vi "Get TDMS channel with scaling.vi"(6 "Samples per read":i64=1000000, 7 "Clip/desimate":T1={"Clip time"=FALSE, "Tiime 0"=0.0, "Time 1"=0.0, "Maximum data points"=1, "Decimation method"=enum."Min-Max"}, 8 "error in":errorcluster, 9 "Channel name":string, 10 "group name":string, 11 "tdms file":refnum<k34>) -> (0 "error out":errorcluster, 1 "output waveform":waveform(dbl), 3 "tdms file out":refnum<k34>)   [LabVIEW 2015]
uses:
  Controls/Data reduction.ctl
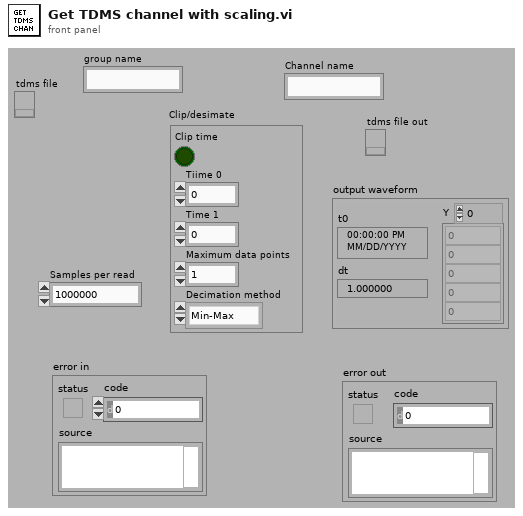
[diagram p1: front panel]
types:
  T1 = typedef "Data reduction.ctl" = cluster{"Clip time":bool, "Tiime 0":dbl, "Time 1":dbl, "Maximum data points":i32, "Decimation method":enum16{"coerce", "linear", "spline", "Min-Max", "Average"}}
  T2 = enum16{"coerce", "linear", "spline", "Min-Max", "Average"}
  T3 = typedef "TDMS channel info.ctl" = cluster{"t0":timestamp, "dt":dbl, "Channel length":i64}
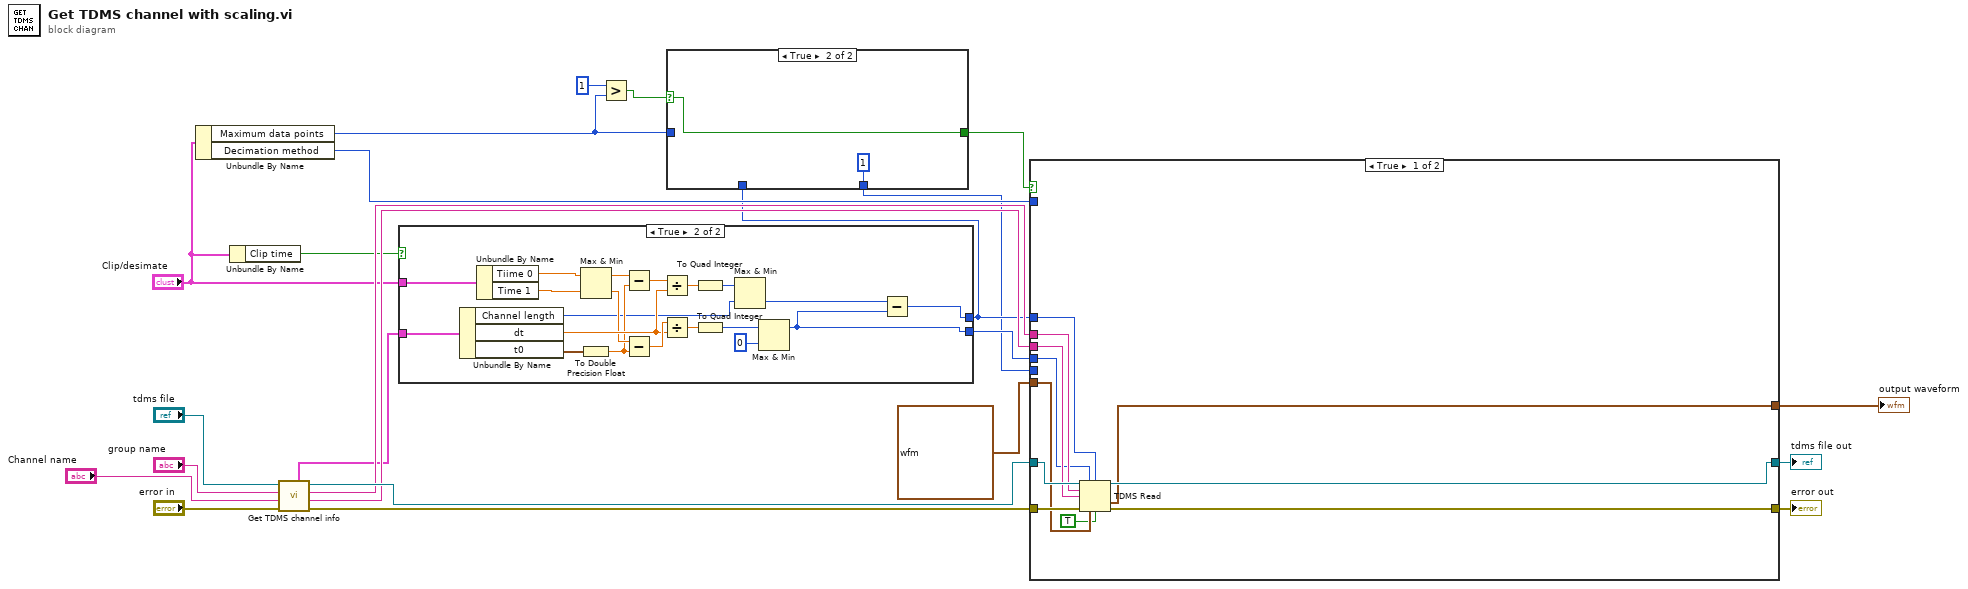
[diagram p0: block diagram]
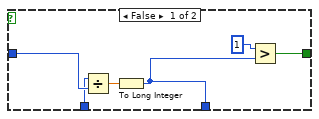
[diagram p2: hidden frame]
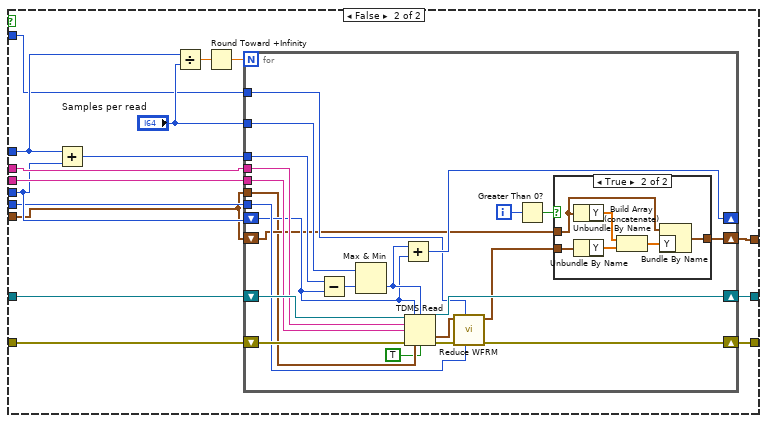
[diagram p3: hidden frame]
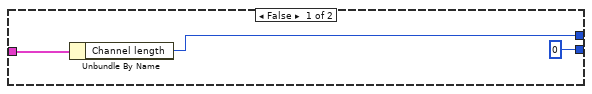
[diagram p5: hidden frame]
diagram:
  n1 = Unbundle By Name("Clip/desimate") -> ("Maximum data points"=w2:i32, "Decimation method"=w10:T2)
  n2 = Unbundle By Name("Clip/desimate") -> ("Clip time"=w7:bool)
  n3 = call "Get TDMS channel info.vi"("error in"="error in", "Channel name"="Channel name", "group name"="group name", "tdms file"="tdms file") -> ("error out"=w19:errorcluster, "channel name out"=w16:string, "group name out"=w17:string, "tdms file out"=w18:refnum<k34>, "TDMS channel info"=w6:T3)  [unwired: 3 in]
  n4 = case shown="True" w7 {
    tunnel: w6 -> [w25 w46]
    tunnel: [i64 0 ("offset (0)") w29] -> w13
    tunnel: [w24 w28] -> w4
    tunnel: "Clip/desimate" -> [_ w37]
    frame False {
      n5 = Unbundle By Name(w25) -> ("Channel length"=w24:i64)
    }
    frame True {
      n6 = Unbundle By Name(w46) -> ("Channel length"=w27:i64, "dt"=w38:dbl, "t0"=w33:timestamp)
      n7 = Unbundle By Name(w37) -> ("Tiime 0"=w36:dbl, "Time 1"=w35:dbl)
      n8 = Max & Min(x=w36, y=w35) -> (max(x,y)=w34:dbl, min(x,y)=w32:dbl)
      n9 = To Double Precision Float(number=w33) -> (double precision float=w31:dbl)
      n10 = Subtract(x=w34, y=w31) -> (x-y=w45:dbl)
      n11 = Subtract(x=w32, y=w31) -> (x-y=w44:dbl)
      n12 = Divide(x=w45, y=w38) -> (x/y=w43:dbl)
      n13 = Divide(x=w44, y=w38) -> (x/y=w40:dbl)
      n14 = To Quad Integer(1:w43) -> (0:w42:i64)
      n15 = To Quad Integer(1:w40) -> (0:w41:i64)
      n16 = Max & Min(x=w42, y=w27) -> (min(x,y)=w30:i64)  [unwired: 1 out]
      n17 = Max & Min(x=w41, y=i64 0) -> (max(x,y)=w29:i64)  [unwired: 1 out]
      n18 = Subtract(x=w30, y=w29) -> (x-y=w28:i64)
    }
  }
  n19 = Greater?(x=1 ("y"), y=w2) -> (0:w5:bool)
  n20 = case shown="True" w5 {
    selector: w5 -> [_ w54]
    tunnel: [w52 w54] -> w12
    tunnel: w2 -> [w49 _]
    tunnel: w4 -> [w48 _]
    tunnel: [w47 1] -> w1
    frame False {
      n21 = Divide(x=w48, y=w49) -> (x/y=w50:dbl)
      n22 = To Long Integer(number=w50) -> (32bit integer=w47:i32)
      n23 = Greater?(x=1 ("y"), y=w47) -> (0:w52:bool)
    }
    frame True {
    }
  }
  n24 = case shown="True" w12 {
    tunnel: w19 -> [w65 w81]
    tunnel: w18 -> [w64 w80]
    tunnel: w17 -> [w63 w79]
    tunnel: w16 -> [w62 w78]
    tunnel: [w61 w77] -> w15
    tunnel: [w60 w76] -> w14
    tunnel: w13 -> [w59 w72]
    tunnel: w4 -> [w58 w71]
    tunnel: [w57 w75] -> w11
    tunnel: w1 -> [_ w69]
    tunnel: w10 -> [_ w67]
    tunnel: waveform(dbl) {"t0"=timestamp(0 s since 1904-01-01), "dt"=1.0, "Y"=[]} ("Waveform out") -> [w56 w66]
    frame True {
      n25 = TDMS Read(0:w64, 1:w59, 2:w58, 5:w63, 7:w62, 11:w65, 12:w56, 13:TRUE ("return channels in file order? (F)")) -> (4:w61:refnum<k34>, 10:w57:waveform(dbl), 15:w60:errorcluster)  [unwired: 3 out]
    }
    frame False {
      n26 = Add(x=w71, y=w72) -> (x+y=w70:i64)
      n27 = Divide(x=w71, y="Samples per read") -> (x/y=w74:dbl)
      n28 = Round Toward +Infinity(x=w74) -> (ceil(x): smallest int >= x=w68:dbl)
      n29 = for {
        N: w68 -> [_]
        tunnel: w79 -> [w102]
        tunnel: w78 -> [w101]
        shift-right: [w100] -> w77
        shift-left: w80 -> [w103]
        shift-right: [w89] -> w76
        shift-left: w81 -> [w104]
        shift-right: [w91] -> _
        shift-left: w72 -> [w92]
        tunnel: "Samples per read" -> [w99]
        tunnel: w70 -> [w98]
        tunnel: w69 -> [w94]
        shift-right: [w88] -> w75
        shift-left: w66 -> [w84]
        tunnel: w67 -> [w87]
        tunnel: w66 -> [w83]
        i -> [w86]
        n30 = Subtract(x=w98, y=w92) -> (x-y=w97:i64)
        n31 = Max & Min(x=w99, y=w97) -> (min(x,y)=w93:i64)  [unwired: 1 out]
        n32 = Add(x=w93, y=w92) -> (x+y=w91:i64)
        n33 = TDMS Read(0:w103, 1:w92, 2:w93, 5:w102, 7:w101, 11:w104, 12:w83, 13:TRUE ("return channels in file order? (F)")) -> (4:w100:refnum<k34>, 10:w95:waveform(dbl), 15:w96:errorcluster)  [unwired: 3 out]
        n34 = call "Reduce WFRM.vi"("decimation factor"=w94, "Decimation method"=w87, "error in (no error)"=w96, "Waveform"=w95) -> ("error out"=w89:errorcluster, "Waveform out"=w90:waveform(sgl))  [unwired: 6 in]
        n35 = Greater Than 0?(x=w86) -> (x > 0?=w85:bool)
        n36 = case shown="True" w85 {
          tunnel: w90 -> [w105 w107]
          tunnel: [w105 w108] -> w88
          tunnel: w84 -> [_ w106]
          frame False {
          }
          frame True {
            n37 = Unbundle By Name(w106) -> ("Y"=w110:dbl[])
            n38 = Unbundle By Name(w107) -> ("Y"=w111:sgl[])
            n39 = Build Array (concatenate)(w110, w111) -> (w109:dbl[])
            n40 = Bundle By Name(cluster=w106, "Y"=w109) -> (w108:waveform(dbl))
          }
        }
      }
    }
  }
  "tdms file out" <- w15
  "error out" <- w14
  "output waveform" <- w11
